vi "collectLT_img_v2.vi"(2 "stream?":bool, 3 "data file":path=path "C:/Users/Labmember/Desktop/Data/temp" caption="data dir.") -> (0 "cts/sec":dbl, 1 "total counts":i32)   [LabVIEW 2015]
uses:
  phlib.dll
panel:
  out "acq time":i32
  out "Fifo overrun":bool
  out "buffer size":i32
  out "exp iterations":i32=5
  out "counts per\niteration":i32[](array[numeric])
  out "trunc buffer":u32[](array[numeric]) format="%08x"
  out "buffer":u32[](array[numeric]) format="%08x"
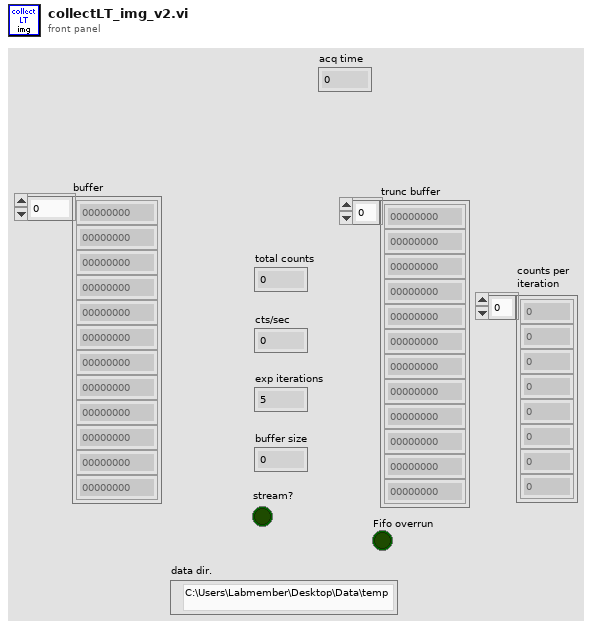
[diagram p1: front panel]
types:
  T1 = enum16{"open", "replace", "create", "open or create", "replace or create", "replace or create with confirmation"}
  T2 = typedef "LVRectTypeDef.ctl" = cluster{"Left":i16, "Top":i16, "Right":i16, "Bottom":i16}
  T3 = cluster{"Xpixels":i32, "Vxminref":dbl, "Vxmaxref":dbl, "P":dbl, "Ypixels":i32, "Vyminref":dbl, "Vymaxref":dbl, "srate":sgl, "sAOxy":i32, "timeout":dbl, "type":string, "date":string, "time":string, "Colormap":u16, "Drawing Mode":u16, "Scanning Mode":u16, "square pixels":bool, "square matrix":bool, "Xpixels Img":i32, "Vx-min Img":dbl, "VX-max Img":dbl, "Ypixels Img":i32, "Vy-min Img":dbl, "Vy-max Img ":dbl, "Angle Img":dbl, "autoshutter":bool, "finite":bool, "cont":bool, "wavdet":bool, "measpoints":i32, "avpp":i32, "bufferAO":i32, "bufferAI":i32, "starttick":u32, "waveform":path, "Vx-ref":dbl, "Vy-ref":dbl, "refreshrate":dbl, "refreshbuffer":i32, "tt_cycles":i32, "motorref":refnum<k7>, "mirrorswitch":refnum<k7>, "sample mode":i32, "maxbufferAI":i32, "srateAODO":sgl, "bin":sgl, "Pel":sgl, "Angle draw":dbl, "srate Img":sgl, "ROIimg_plotbounds":T2, "auto OD":bool, "ODfilt":u16, "aAI":i32[], "aCI":i32[], "aAO":u32[], "aDO":u32[], "refwfsize":dbl, "Lifetime":bool, "Vz-Img":dbl, "Vz-ref":dbl, "Vz-reset":dbl, "AIoverride":bool, "aAS":u32[], "XYZstart":dbl[]}
  T4 = cluster{"initialized":bool, "devidx":i32, "Ch0 Level":i32, "Ch0 ZeroX":i32, "Ch1 Level":i32, "Ch1 ZeroX":i32, "sync rate":i32, "resolution":i32, "acq time":i32, "acq rate":i32, "# bins":u32, "Bin size":enum16{"1", "2", "4", "8", "16", "32", "64", "128"}, "min photons":u32, "truncate":u32}
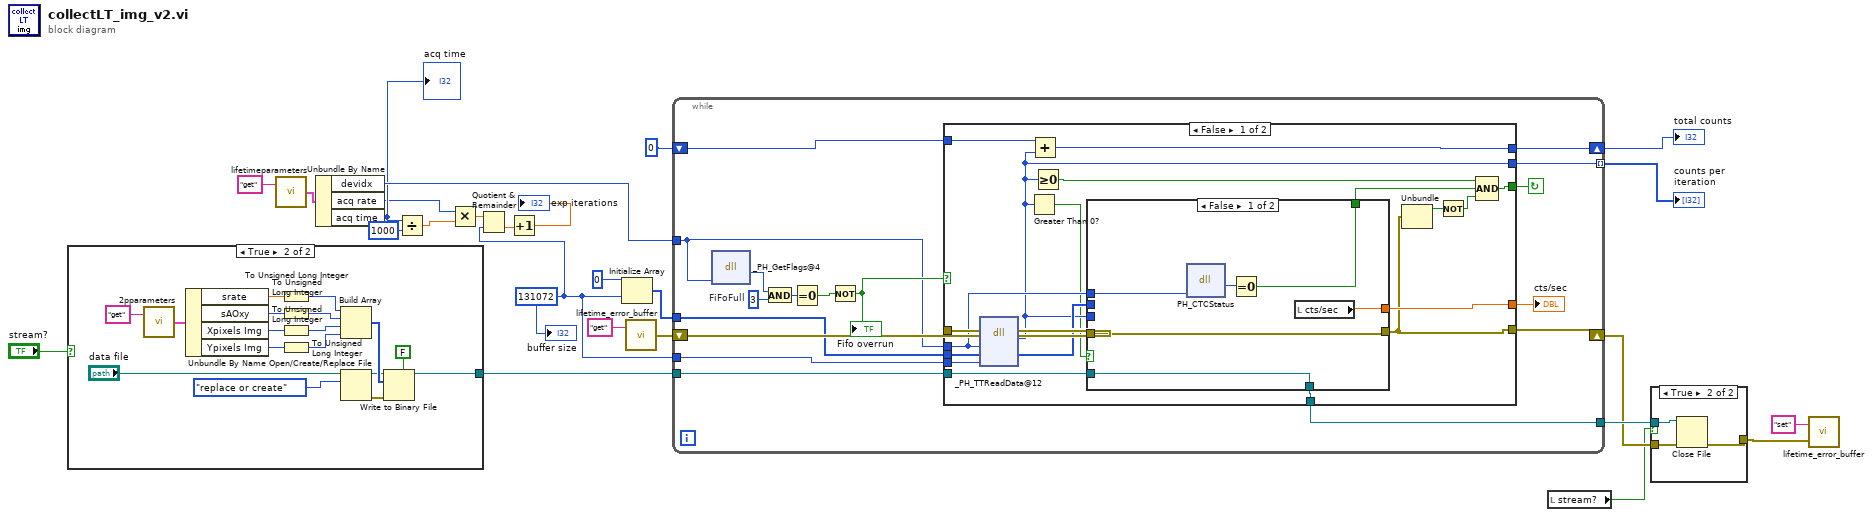
[diagram p0: block diagram]
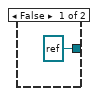
[diagram p3: hidden frame]
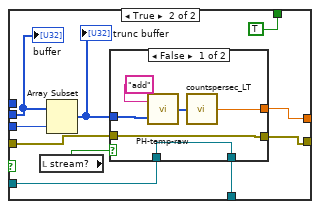
[diagram p4: hidden frame]
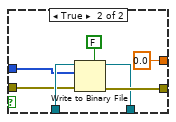
[diagram p5: hidden frame]
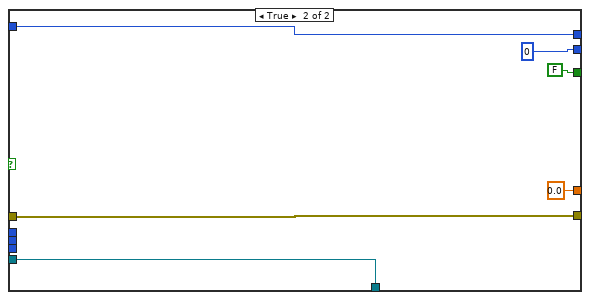
[diagram p6: hidden frame]
diagram:
  w11 = 131072 ("y")
  n1 = case shown="True" "stream?" {
    tunnel: [refnum<file> refnum ("refnum out") w29] -> w7
    frame False {
    }
    frame True {
      n2 = call "2pparameters.vi"("command"="get") -> ("params out"=w41:T3)  [unwired: 1 in]
      n3 = Unbundle By Name(w41) -> ("srate"=w39:sgl, "sAOxy"=w38:i32, "Xpixels Img"=w36:i32, "Ypixels Img"=w34:i32)
      n4 = To Unsigned Long Integer(number=w39) -> (unsigned 32bit integer=w40:u32)
      n5 = To Unsigned Long Integer(number=w38) -> (unsigned 32bit integer=w37:u32)
      n6 = To Unsigned Long Integer(number=w36) -> (unsigned 32bit integer=w35:u32)
      n7 = To Unsigned Long Integer(number=w34) -> (unsigned 32bit integer=w33:u32)
      n8 = Build Array(w40, w37, w35, w33) -> (w32:u32[])
      n9 = Open/Create/Replace File(file path (use dialog)="data file", operation (0:open)=T1."replace or create") -> (refnum out=w31:refnum<file>, error out=w30:errorcluster)  [unwired: 4 in, 1 out]
      n10 = Write to Binary File(file (use dialog)=w31, data=w32, error in=w30, 5:FALSE ("prepend array or string size? (T)")) -> (refnum out=w29:refnum<file>)  [unwired: 2 in, 2 out]
    }
  }
  n11 = call "lifetimeparameters.vi"("command"="get") -> ("Params out"=w22:T4)  [unwired: 1 in]
  n12 = Unbundle By Name(w22) -> ("devidx"=w21:i32, "acq rate"=w12:i32, "acq time"=w13:i32)
  "acq time" <- w13
  n13 = Divide(x=w13, y=1000) -> (x/y=w1:dbl)
  n14 = Multiply(x=w12, y=w1) -> (x*y=w10:dbl)
  n15 = Quotient & Remainder(x=w10, y=w11) -> (floor(x/y)=w14:dbl)  [unwired: 1 out]
  n16 = Increment(x=w14) -> (x+1=→"exp iterations":dbl)
  n17 = Initialize Array(u32 0, w11) -> (w17:u32[])
  n18 = call "lifetime_error_buffer.vi"("command"="get") -> ("error out"=w24:errorcluster)  [unwired: 1 in]
  n19 = while {
    tunnel: w21 -> [w46]
    shift-right: [w59] -> w5
    shift-left: w24 -> [w60]
    tunnel: [w56] -> w19 mode=indexing
    tunnel: w17 -> [w58]
    tunnel: w11 -> [w57]
    shift-right: [w55] -> w16
    shift-left: 0 ("return type") -> [w54]
    tunnel: w7 -> [w45]
    tunnel: [w44] -> w6
    stop <- w48 continue-if-true
    w50 = 3  # FiFoFull
    n20 = dll-call lib="phlib.dll" fn="_PH_GetFlags@4" label="PH_GetFlags"("devidx"=w46) -> (w52:i32)  [unwired: 4 in, 2 out]
    n21 = And(x=w52, y=w50) -> (x .and. y?=w51:i32)
    n22 = Equal To 0?(x=w51) -> (x = 0?=w53:bool)
    n23 = Not ("CTCDone")(x=w53) -> (.not. x?=w49:bool)
    "Fifo overrun" <- w49
    n24 = case shown="False" w49 {
      tunnel: w60 -> [w79 w112]
      tunnel: [w68 w112] -> w59
      tunnel: w46 -> [w73 _]
      tunnel: w58 -> [w78 _]
      tunnel: w57 -> [w77 _]
      tunnel: [w62 0 ("return type")] -> w56
      tunnel: [w76 w111] -> w55
      tunnel: w54 -> [w75 w111]
      tunnel: [w63 FALSE] -> w48
      tunnel: [w71 0.0 ("Avg cts/s")] -> w47
      tunnel: w45 -> [w70 w109]
      tunnel: [w69 w109] -> w44
      frame False {
        n25 = dll-call lib="phlib.dll" fn="_PH_TTReadData@12" label="PH_TTReadData"(error in=w79, "devidx"=w73, "buffer"=w78, "blocksize"=w77) -> (error out=w74:errorcluster, "return type"=w62:i32, "buffer"=w72:u32[])  [unwired: 4 in, 1 out]
        n26 = Greater Than 0?(x=w62) -> (x > 0?=w61:bool)
        n27 = Add(x=w75, y=w62) -> (x+y=w76:i32)
        n28 = Greater Or Equal To 0?(x=w62) -> (x >= 0?=w64:bool)
        n29 = case shown="False" w61 {
          tunnel: [w85 w88] -> w68
          tunnel: w74 -> [w85 w89]
          tunnel: [w83 TRUE] -> w65
          tunnel: w73 -> [w82 _]
          tunnel: w72 -> [_ w94]
          tunnel: w62 -> [_ w93]
          tunnel: [w81 w92] -> w71
          tunnel: w70 -> [w80 w90]
          tunnel: [w80 w86] -> w69
          frame False {
            n30 = dll-call lib="phlib.dll" fn="PH_CTCStatus"("devidx"=w82) -> (w84:i32)  [unwired: 4 in, 2 out]
            n31 = Equal To 0?(x=w84) -> (x = 0?=w83:bool)
            n32 = local read "cts/sec"() -> (w81:dbl)
          }
          frame True {
            n33 = local read "stream?"() -> (w87:bool)
            n34 = Array Subset(array=w94, length=w93) -> (w95:u32[])  [unwired: 1 in]
            "trunc buffer" <- w95
            n35 = case shown="False" w87 {
              tunnel: w95 -> [w100 w105]
              tunnel: [w98 0.0 ("Avg cts/s")] -> w92
              tunnel: w90 -> [w96 w106]
              tunnel: w89 -> [w97 w104]
              tunnel: [w97 w103] -> w88
              tunnel: [w96 w102] -> w86
              frame False {
                n36 = call "PH-temp-raw.vi"("array in"=w100, "command"="add") -> ("array out"=w101:u32[])
                n37 = call "countspersec_LT.vi"("1D PH data"=w101) -> ("Avg cts/s"=w98:dbl)
              }
              frame True {
                n38 = Write to Binary File(file (use dialog)=w106, data=w105, error in=w104, 5:FALSE ("prepend array or string size? (T)")) -> (refnum out=w102:refnum<file>, error out=w103:errorcluster)  [unwired: 2 in, 1 out]
              }
            }
            "buffer" <- w94
          }
        }
        n39 = Unbundle(w68) -> ("status"=w67:bool)  [unwired: 2 out]
        n40 = Not(x=w67) -> (.not. x?=w66:bool)
        n41 = Compound Arithmetic op=AND(w64, w65, w66) -> (w63:bool)
      }
      frame True {
      }
    }
    "cts/sec" <- w47
  }
  "counts per\niteration" <- w19
  "total counts" <- w16
  n42 = local read "stream?"() -> (w3:bool)
  n43 = case shown="True" w3 {
    tunnel: w6 -> [_ w118]
    tunnel: w5 -> [w115 w117]
    tunnel: [w115 w116] -> w4
    frame False {
    }
    frame True {
      n44 = Close File(refnum=w118, error in=w117) -> (error out=w116:errorcluster)  [unwired: 1 out]
    }
  }
  n45 = call "lifetime_error_buffer.vi"("error in"=w4, "command"="set") -> ()  [unwired: 1 out]
  "buffer size" <- w11
